vi "SetVoltage.vi"(8 "error in (no error)":errorcluster, 10 "Voltage":dbl, 11 "TecellaChannel in":refnum<class "TecellaChannel.lvclass">) -> (0 "error out":errorcluster, 3 "TecellaChannel out":refnum<class "TecellaChannel.lvclass">)   [LabVIEW 2009, in "TecellaChannel.lvclass"]
uses:
  TecellaChannel.lvclass
  TecellaChannel.lvclass/TecellaChannel.ctl
  TecellaClient/TecellaClient.lvclass
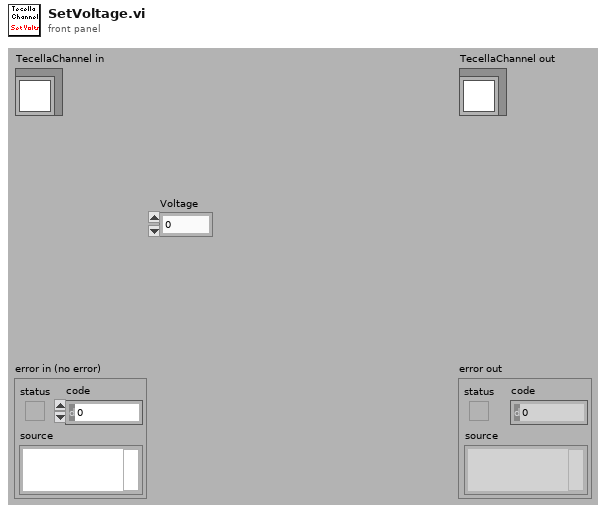
[diagram p1: front panel]
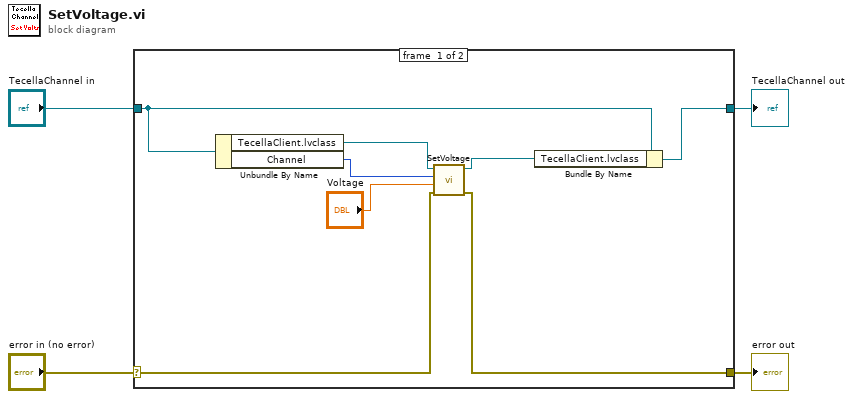
[diagram p0: block diagram]
diagram:
  n1 = case shown="No Error" "error in (no error)" {
    selector: "error in (no error)" -> [w7 w14]
    tunnel: [w6 w14] -> w3
    tunnel: [w11 w13] -> w1
    tunnel: "TecellaChannel in" -> [w12 w13]
    frame #0 {
      n2 = Unbundle By Name(w12) -> ("TecellaClient.lvclass"=w9:refnum<class "TecellaClient.lvclass">, "Channel"=w10:i8)
      n3 = call-dynamic "SetVoltage.vi"("error in (no error)"=w7, "Voltage"="Voltage", "Channel"=w10, "TecellaClient in"=w9) -> ("error out"=w6:errorcluster, "TecellaClient out"=w5:refnum<class "TecellaClient.lvclass">)  [unwired: 6 in]
      n4 = Bundle By Name(cluster=w12, "TecellaClient.lvclass"=w5) -> (w11:refnum<class "TecellaChannel.lvclass">)
    }
    frame #1 {
    }
  }
  "error out" <- w3
  "TecellaChannel out" <- w1
